vi "LEBITplc.Selector.vi"(0 "i ref in":refnum<vi>, 2 "selector in":string) -> (14 "i ref out":refnum<vi>, 15 "Nickname":string, 16 "index of element":i32, 17 "Special Data":string, 18 "selector out":string)   [LabVIEW 2014, in "LEBITplc.lvlib"]
uses:
  LEBITplc.lvlib
panel:
  out "error out":errorcluster
  in  "error in (no error)":errorcluster
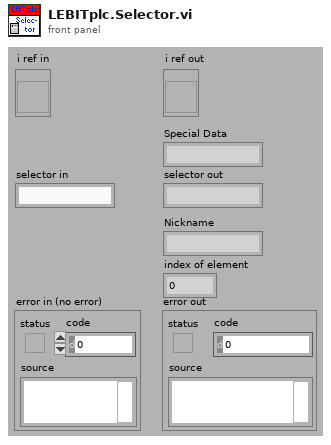
[diagram p1: front panel]
types:
  T1 = typedef "LEBITplc.lvlib/LEBITplc.i attribute.ctl" = cluster{"LLFLocation":string, "SetFileLocation":string, "nickNames":string[], "setValuePLCServiceID":i32[], "GUIServiceID":i32[], "monValuePLC":string[], "SetValueServiceID":i32[], "MonValueServiceID":i32[], "SetValue":dbl[][], "SetValueMin":dbl[], "SetValueMax":dbl[], "SetValueInfoServiceID":i32[], "GUINames":string[], "ListOfBases":string[], "Scale":dbl[], "Offset":dbl[], "setValuePLC":string[], "BaseName":string[], "ScaleServiceID":i32[], "OffsetServiceID":i32[], "AllPLCValues":string[], "CondSpecialArray":string[][], "CondSpecialIndex":i32[], "CondSpecialMonValue":dbl[], "RecentlyChanged":i32[], "SetFileLocationID":i32, "Dependent-Monitors":string[][], "LastLoadedFiles":string[], "IonGuideCalibLocation":string, "Monitor Dependent":string[], "Special":string[], "PLC?":bool[], "Start Date":string, "ListOfBasesServiceID":i32, "SETRA VISA resource":refnum<visa-resource-name>}
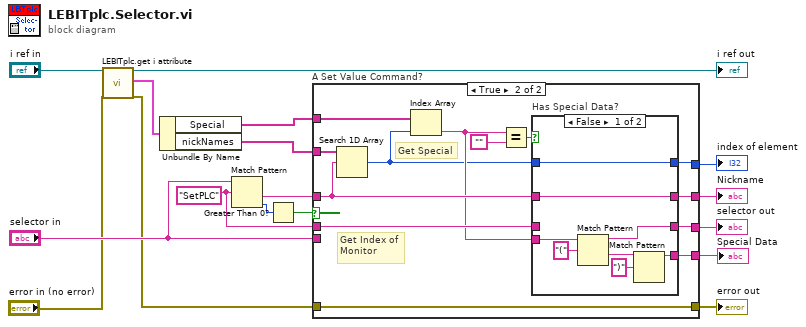
[diagram p0: block diagram]
diagram:
  w6 = "SetPLC" ("regular expression")
  n1 = call "LEBITplc.get i attribute.vi"("i ref in"="i ref in", "error in (no error)"="error in (no error)") -> ("i ref out"=→"i ref out":refnum<vi>, "i attribute"=w12:T1, "error out"=w3:errorcluster)  [unwired: 15 in]
  n2 = Unbundle By Name(w12) -> ("Special"=w4:string[], "nickNames"=w5:string[])
  n3 = Match Pattern(string="selector in", regular expression=w6) -> (after substring=w7:string, offset past match=w9:i32)  [unwired: 1 in, 2 out]
  n4 = Greater Than 0?(x=w9) -> (x > 0?=w8:bool)
  n5 = case "A Set Value Command?" shown="True" w8 {
    tunnel: w7 -> [_ w27]
    tunnel: [_ w28] -> w11
    tunnel: [w19 w23] -> w13
    tunnel: "selector in" -> [w19 _]
    tunnel: w6 -> [_ w25]
    tunnel: w5 -> [_ w32]
    tunnel: [_ w29] -> w10
    tunnel: w4 -> [_ w30]
    tunnel: [w18 w22] -> w2
    tunnel: w3 -> [w18 w22]
    tunnel: [_ w21] -> w1
    frame False {
    }
    frame True {
      # "Get Special"
      # "Get Index of\nMonitor"
      n6 = Search 1D Array(1D array=w32, element=w27) -> (index of element=w20:i32)  [unwired: 1 in]
      n7 = Index Array(array=w30, index=w20) -> (element=w24:string)
      n8 = Equal?(x=w24, y="") -> (x = y?=w26:bool)
      n9 = case "Has Special Data?" shown="False" w26 {
        tunnel: w20 -> [w40 w43]
        tunnel: [w40 w43] -> w29
        tunnel: [w39 w42] -> w28
        tunnel: w27 -> [w39 w42]
        tunnel: w25 -> [_ w41]
        tunnel: w24 -> [w37 _]
        tunnel: [w35 w41] -> w23
        tunnel: [w33 _] -> w21
        frame False {
          n10 = Match Pattern(string=w37, regular expression="(") -> (before substring=w35:string, after substring=w34:string)  [unwired: 1 in, 2 out]
          n11 = Match Pattern(string=w34, regular expression=")") -> (before substring=w33:string)  [unwired: 1 in, 3 out]
        }
        frame True {
        }
      }
    }
  }
  "Nickname" <- w11
  "selector out" <- w13
  "index of element" <- w10
  "error out" <- w2
  "Special Data" <- w1
